vi "Combine 3D Point Sets.vi"(8 "error in":errorcluster, 11 "Point Sets in":map{i32, T1}[](array[numeric])) -> (0 "error out":errorcluster, 1 "Discarded":map{i32, T1}[](array[numeric]), 3 "Combined Point Set":map{i32, T1}(c390))   [LabVIEW 2020, in "ar.lvlib"]
doc: "Combine multiple 3D Point Sets. The Point Sets must have sufficient overlap to allow them to be combined."
uses:
  ar.lvlib
  common/Object Point (Float).ctl
  <vilib>/Analysis/baseanly.llb/A x Vector.vi
  common/common.lvlib
  <vilib>/Analysis/Matrix/NI_Matrix.lvlib
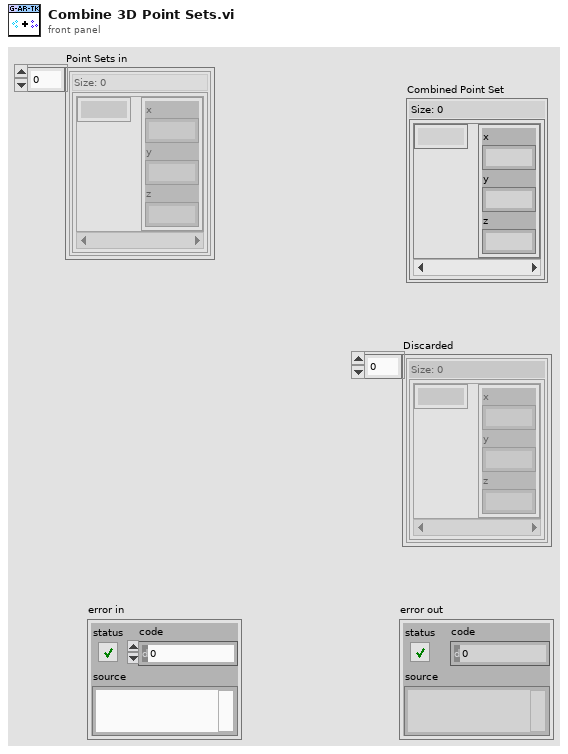
[diagram p1: front panel]
types:
  T1 = typedef "common.lvlib/Object Point (Float).ctl" = cluster{"x":dbl, "y":dbl, "z":dbl}
  T2 = typedef "NI_Matrix.lvlib/RealMatrix.ctl" = dbl[][]
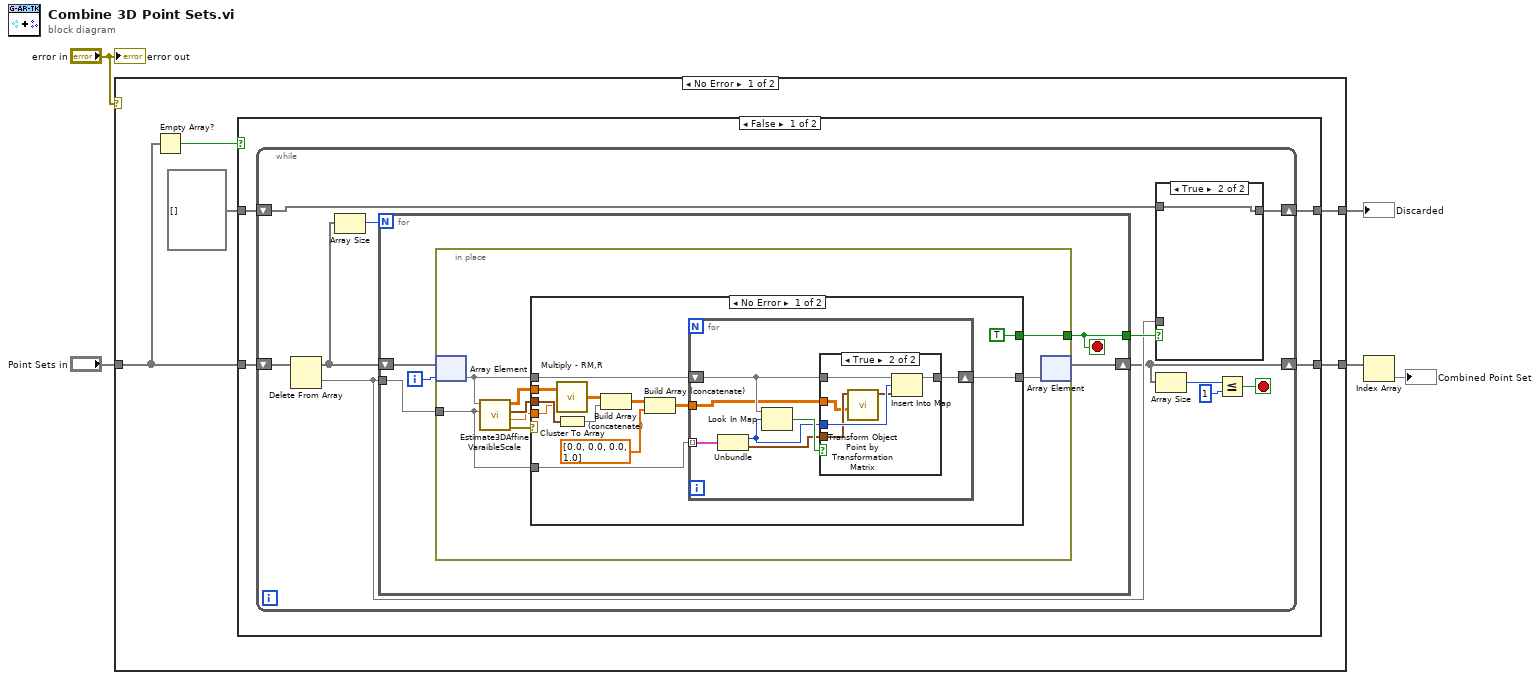
[diagram p0: block diagram]
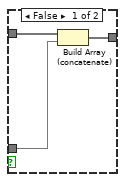
[diagram p2: hidden frame]
diagram:
  n1 = case shown="No Error" "error in" {
    tunnel: [w10 _] -> w5
    tunnel: [w8 _] -> w2
    tunnel: "Point Sets in" -> [w7 _]
    frame No Error {
      n2 = Empty Array?(array=w7) -> (empty?=w6:bool)
      n3 = case shown="False" w6 {
        tunnel: [w14 w70] -> w10
        tunnel: map{i32, T1}[] [] -> [w13 w70]
        tunnel: [w12 w71] -> w8
        tunnel: w7 -> [w11 w71]
        frame False {
          n4 = while {
            shift-right: [w16] -> w12
            shift-left: w11 -> [w25]
            shift-right: [w17] -> w14
            shift-left: w13 -> [w19]
            stop <- w15 stop-if-true
            n5 = Delete From Array(array=w25) -> (deleted portion=w18:map{i32, T1}, array with subset deleted=w21:map{i32, T1}[])  [unwired: 2 in]
            n6 = Array Size(array=w21) -> (size(s)=w22:i32)
            n7 = for {
              N: w22 -> [_]
              tunnel: w18 -> [w32]
              shift-right: [w30] -> w16
              shift-left: w21 -> [w34]
              tunnel: [w31] -> w20
              i -> [w33]
              stop <- w31 stop-if-true
              n8 = in-place {
                in-place-border: w32 -> [w37]
                in-place-border: [w38] -> w31
                n9 = in-place-array #1(w34, w33) -> (w36:map{i32, T1})
                n10 = call "Estimate3DAffineVaraibleScale.vi"("To"=w37, "From"=w36) -> ("error out"=w40:errorcluster, "Scale"=w35:dbl, "T"=w42:T1, "R"=w41:T2)  [unwired: 6 in]
                n11 = case shown="No Error" w40 {
                  tunnel: [w49 w69] -> w39
                  tunnel: w36 -> [w51 w69]
                  tunnel: w37 -> [w50 _]
                  tunnel: w41 -> [w45 _]
                  tunnel: w42 -> [w54 _]
                  tunnel: [TRUE _] -> w38
                  tunnel: w35 -> [w43 _]
                  frame No Error {
                    n12 = call <vilib>:"Multiply - RM,R.vi"("Real Scalar c"=w43, "Real Matrix A"=w45) -> ("A * c"=w44:T2)
                    n13 = Cluster To Array(cluster=w54) -> (array=w53:dbl[])
                    n14 = Build Array (concatenate)(w44, w53) -> (w52:T2)
                    n15 = Build Array (concatenate)(w52, dbl[] [0.0, 0.0, 0.0, 1.0]) -> (w46:T2)
                    n16 = for {
                      shift-right: [w59] -> w49
                      shift-left: w51 -> [w58]
                      tunnel: w50 -> [w61] mode=indexing
                      tunnel: w46 -> [w55]
                      n17 = Unbundle(w61) -> ("Index"=w57:i32, "Object Point"=w56:T1)
                      n18 = Look In Map(map=w58, key=w57) -> (key not found?=w60:bool)  [unwired: 1 in, 1 out]
                      n19 = case shown="True" w60 {
                        tunnel: [w62 w67] -> w59
                        tunnel: w58 -> [w62 w68]
                        tunnel: w57 -> [_ w66]
                        tunnel: w56 -> [_ w65]
                        tunnel: w55 -> [_ w64]
                        frame False {
                        }
                        frame True {
                          n20 = call "Transform Object Point by Transformation Matrix.vi"("Transformation Matrix (4x4)"=w64, "Object Point"=w65) -> ("Transformed Point"=w63:T1)  [unwired: 8 in, 1 out]
                          n21 = Insert Into Map(map in=w68, key=w66, value=w63) -> (map out=w67:map{i32, T1})  [unwired: 2 out]
                        }
                      }
                    }
                  }
                  frame Error {
                  }
                }
                n22 = in-place-array #1(w39) -> (w30:map{i32, T1}[])  [unwired: 1 out]
              }
            }
            n23 = case shown="True" w20 {
              tunnel: w19 -> [w28 w29]
              tunnel: w18 -> [w27 _]
              tunnel: [w26 w29] -> w17
              frame False {
                n24 = Build Array (concatenate)(w28, w27) -> (w26:map{i32, T1}[])
              }
              frame True {
              }
            }
            n25 = Array Size(array=w16) -> (size(s)=w24:i32)
            n26 = Less Or Equal?(x=w24, y=1) -> (x <= y?=w15:bool)
          }
        }
        frame True {
        }
      }
    }
    frame Error {
    }
  }
  "Discarded" <- w5
  n27 = Index Array(array=w2) -> (element=→"Combined Point Set":map{i32, T1})  [unwired: 1 in]
  "error out" <- "error in"
